vi "DataGraph_Clear_SelRange_Plot.vi"(1 "reference in":refnum<vi>) -> (0 "reference out":refnum<vi>)   [LabVIEW 2018, in "DataGraphXControl.xctl"]
uses:
  DataGraphXControl.xctl
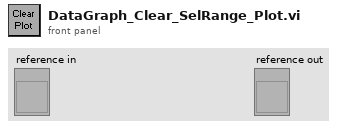
[diagram p1: front panel]
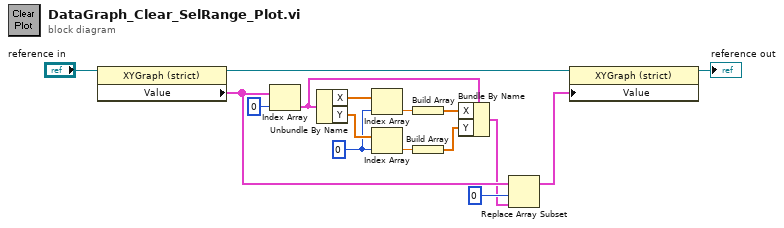
[diagram p0: block diagram]
diagram:
  w13 = 0 ("index")
  n1 = property class="XYGraph (strict)"(reference="reference in") -> (reference out=w4:refnum<vi>, "Value"=w7:cluster{"X":dbl[], "Y":dbl[]}[])  [unwired: 1 in, 1 out]
  n2 = Index Array(array=w7, index=0) -> (element=w12:cluster{"X":dbl[], "Y":dbl[]})
  n3 = Unbundle By Name(w12) -> ("X"=w15:dbl[], "Y"=w14:dbl[])
  n4 = Index Array(array=w15, index=w13) -> (element=w10:dbl)
  n5 = Index Array(array=w14, index=w13) -> (element=w11:dbl)
  n6 = Build Array(w10) -> (w9:dbl[])
  n7 = Build Array(w11) -> (w8:dbl[])
  n8 = Bundle By Name(cluster=w12, "X"=w9, "Y"=w8) -> (w5:cluster{"X":dbl[], "Y":dbl[]})
  n9 = Replace Array Subset(array=w7, new element=w5, index=0) -> (w3:cluster{"X":dbl[], "Y":dbl[]}[])
  n10 = property class="XYGraph (strict)"(reference=w4, "Value"=w3) -> (reference out=→"reference out":refnum<vi>)  [unwired: 1 in, 1 out]
